vi "IP Address -Set.vi"(5 "IP Address":string="192.168.25.3", 7 "Submet Mask":string="255.255.255.0", 11 "error in (no error)":errorcluster) -> (4 "return code":i32, 6 "standard output":string, 8 "standard error":string, 15 "error out":errorcluster)   [LabVIEW 2013]
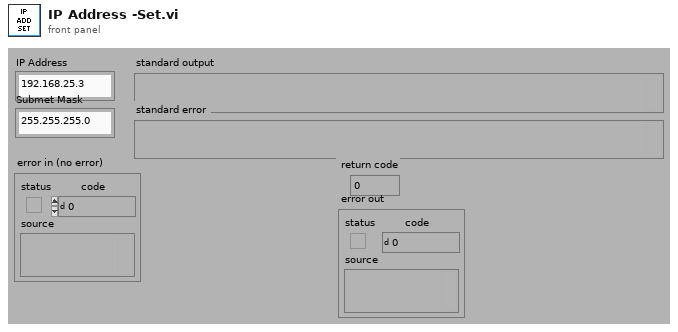
[diagram p1: front panel]
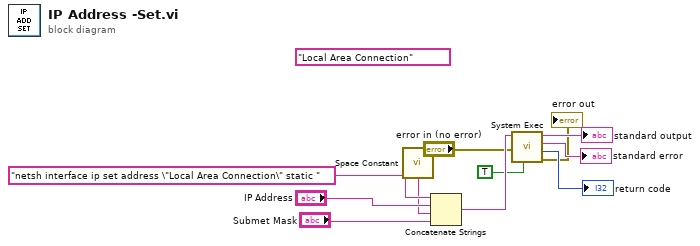
[diagram p0: block diagram]
diagram:
  (unwired) "Local Area Connection" ("command line")
  n1 = call <vilib>:"Space Constant.vi"() -> ("String"=w8:string)
  n2 = Concatenate Strings("netsh interface ip set address \"Local Area Connection\" static " ("command line"), "IP Address", w8, "Submet Mask") -> (w11:string)
  n3 = call <vilib>:"System Exec.vi"("run minimized? (F)"=TRUE, "error in (no error)"="error in (no error)", "command line"=w11) -> ("error out"=→"error out":errorcluster, "return code"=→"return code":i32, "standard error"=→"standard error":string, "standard output"=→"standard output":string)  [unwired: 5 in]
